vi "Set Project Model.vi"(8 "error in (no error)":errorcluster, 10 "Project.lvclass":refnum<class "BrowerComponent.lvclass">, 11 "BrowerController in":refnum<class "BrowerController.lvclass">) -> (0 "error out":errorcluster, 3 "BrowerController out":refnum<class "BrowerController.lvclass">)   [LabVIEW 2015, in "BrowerController.lvclass"]
uses:
  BrowerController.lvclass
  Models/BrowerComponent/BrowerComponent/BrowerComponent.lvclass
  BrowerController.lvclass/BrowerController.ctl
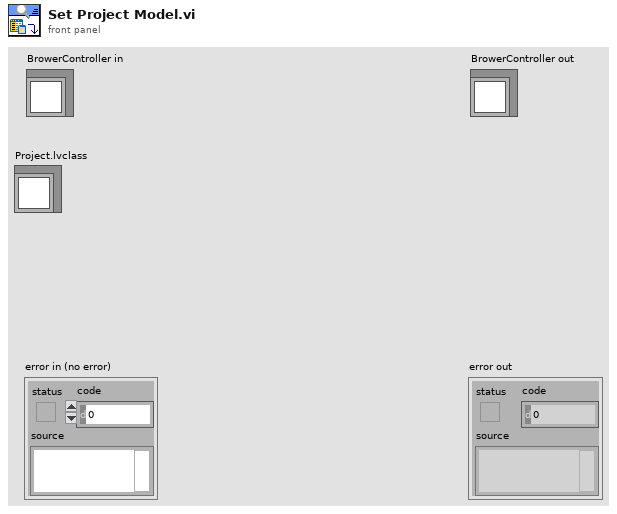
[diagram p1: front panel]
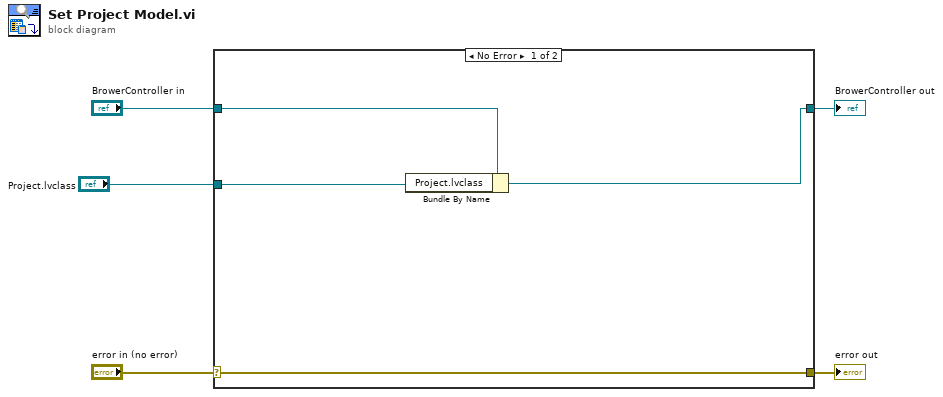
[diagram p0: block diagram]
diagram:
  n1 = case shown="No Error" "error in (no error)" {
    selector: "error in (no error)" -> [w9 w11]
    tunnel: [w9 w11] -> w4
    tunnel: [w7 w10] -> w2
    tunnel: "BrowerController in" -> [w8 w10]
    tunnel: "Project.lvclass" -> [w6 _]
    frame No Error {
      n2 = Bundle By Name(cluster=w8, "Project.lvclass"=w6) -> (w7:refnum<class "BrowerController.lvclass">)
    }
    frame Error {
    }
  }
  "error out" <- w4
  "BrowerController out" <- w2
